vi "StoreArrays_V2.vi"(9 "Numeric":dbl, 10 "Value":u32[](array[numeric]), 11 "Value 2":i32[](array[numeric])) -> (3 "Cluster":cluster{"Value 2":i32[], "Value":u32[]})   [LabVIEW 2020]
uses:
  <vilib>/Utility/NIReport.llb/Report Type.ctl
  <vilib>/addons/_office/excel.llb/Excel Easy Table (str).vi
  <vilib>/Utility/NIReport.llb/NI_report.lvclass
  <vilib>/Utility/NIReport.llb/NI_ReportGenerationCore.lvlib
  <vilib>/Utility/NIReport.llb/Excel/NI_Excel.lvclass
  <vilib>/addons/_office/NI_ReportGenerationToolkit.lvlib
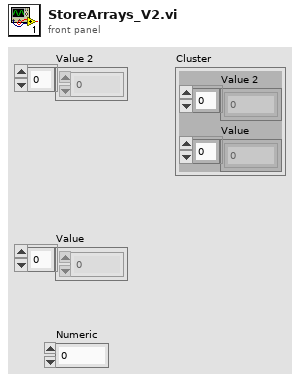
[diagram p1: front panel]
types:
  T1 = enum16{"open", "replace", "create", "open or create", "replace or create", "replace or create with confirmation"}
  T2 = typedef "NI_ReportGenerationCore.lvlib/Report Type.ctl" = enum16{"HTML", "Word", "Excel"}
  T3 = typedef "NI_Matrix.lvlib/RealMatrix.ctl" = dbl[][]
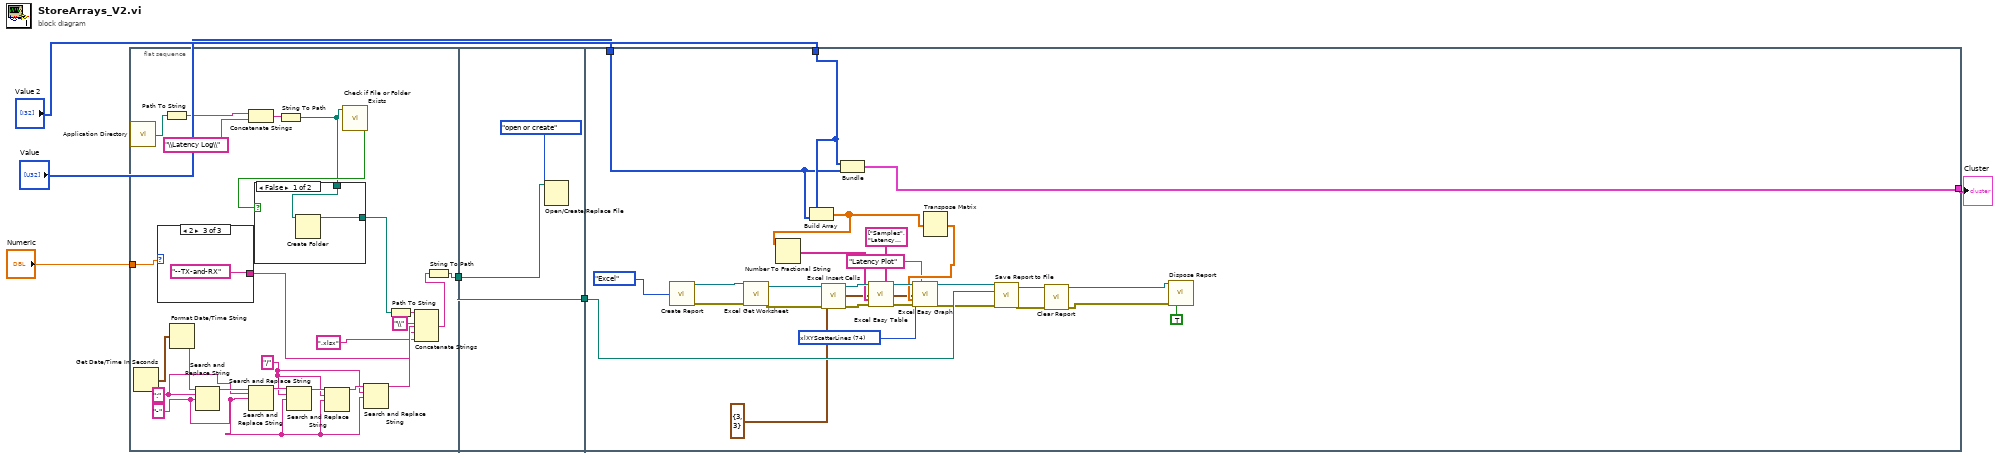
[diagram p0: block diagram]
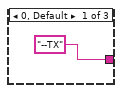
[diagram p2: hidden frame]
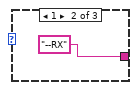
[diagram p3: hidden frame]
diagram:
  n1 = flat-sequence {
    tunnel: [w28] -> w6
    tunnel: "Numeric" -> [w8]
    tunnel: [w37] -> w5
    tunnel: w6 -> [w37]
    tunnel: w5 -> [w61]
    tunnel: "Value 2" -> [w55]
    tunnel: "Value" -> [w54]
    tunnel: [w56] -> w1
    frame #0 {
      w12 = "/" ("search string")
      w11 = "-" ("replace string (\"\")")
      w10 = ":" ("search string")
      n2 = call <vilib>:"Application Directory.vi"() -> ("Application Directory"=w25:path)
      n3 = Get Date/Time In Seconds() -> (seconds since 1Jan1904=w29:timestamp)
      n4 = case shown="2" w8 {
        tunnel: ["--TX" "--RX" "--TX-and-RX"] -> w7
        frame 0, Default {
        }
        frame 1 {
        }
        frame 2 {
        }
      }
      n5 = Path To String(path=w25) -> (string=w26:string)
      n6 = Format Date/Time String(seconds (now)=w29) -> (date/time string=w30:string)  [unwired: 2 in]
      n7 = Search and Replace String(input string=w30, search string=w10, replace string=w11) -> (result string=w17:string)  [unwired: 5 in, 3 out]
      n8 = Concatenate Strings(w26, "\\Latency Log\\" ("string")) -> (w23:string)
      n9 = Search and Replace String(input string=w17, search string=w10, replace string=w11) -> (result string=w16:string)  [unwired: 5 in, 3 out]
      n10 = String To Path(string=w23) -> (path=w19:path)
      n11 = Search and Replace String(input string=w16, search string=w12, replace string=w11) -> (result string=w15:string)  [unwired: 5 in, 3 out]
      n12 = Search and Replace String(input string=w15, search string=w12, replace string=w11) -> (result string=w14:string)  [unwired: 5 in, 3 out]
      n13 = call <vilib>:"Check if File or Folder Exists.vi"("path"=w19) -> ("file or folder exists?"=w22:bool)  [unwired: 8 in, 2 out]
      n14 = case shown="False" w22 {
        tunnel: [w35 w36] -> w20
        tunnel: w19 -> [w34 w36]
        frame False {
          n15 = Create Folder(path (use dialog)=w34) -> (created path=w35:path)  [unwired: 2 in, 2 out]
        }
        frame True {
        }
      }
      n16 = Search and Replace String(input string=w14, search string=w12, replace string=w11) -> (result string=w13:string)  [unwired: 5 in, 3 out]
      n17 = Path To String(path=w20) -> (string=w21:string)
      n18 = Concatenate Strings(w21, "\\" ("string"), w13, w7, ".xlsx" ("string")) -> (w27:string)
      n19 = String To Path(string=w27) -> (path=w28:path)
    }
    frame #1 {
      n20 = Open/Create/Replace File(file path (use dialog)=w37, operation (0:open)=T1."open or create") -> ()  [unwired: 4 in, 3 out]
    }
    frame #2 {
      w41 = 74 items=["xlColumnClustered"=51, "xlColumnStacked"=52, "xlColumnStacked100"=53, "xl3DColumnClustered"=54, "xl3DColumnStacked"=55, "xl3DColumnStacked100"=56, "xlBarClustered"=57, "xlBarStacked"=58, "xlBarStacked100"=59, "xl3DBarClustered"=60, "xl3DBarStacked"=61, "xl3DBarStacked100"=62, "xlLineStacked"=63, "xlLineStacked100"=64, "xlLineMarkers"=65, "xlLineMarkersStacked"=66, "xlLineMarkersStacked100"=67, "xlPieOfPie"=68, "xlPieExploded"=69, "xl3DPieExploded"=70, "xlBarOfPie"=71, "xlXYScatterSmooth"=72, "xlXYScatterSmoothNoMarkers"=73, "xlXYScatterLines"=74, "xlXYScatterLinesNoMarkers"=75, "xlAreaStacked"=76, "xlAreaStacked100"=77, "xl3DAreaStacked"=78, "xl3DAreaStacked100"=79, "xlDoughnutExploded"=80, "xlRadarMarkers"=81, "xlRadarFilled"=82, "xlSurface"=83, "xlSurfaceWireframe"=84, "xlSurfaceTopView"=85, "xlSurfaceTopViewWireframe"=86, "xlBubble"=15, "xlBubble3DEffect"=87, "xlStockHLC"=88, "xlStockOHLC"=89, "xlStockVHLC"=90, "xlStockVOHLC"=91, "xlCylinderColClustered"=92, "xlCylinderColStacked"=93, "xlCylinderColStacked100"=94, "xlCylinderBarClustered"=95, "xlCylinderBarStacked"=96, "xlCylinderBarStacked100"=97, "xlCylinderCol"=98, "xlConeColClustered"=99, "xlConeColStacked"=100, "xlConeColStacked100"=101, "xlConeBarClustered"=102, "xlConeBarStacked"=103, "xlConeBarStacked100"=104, "xlConeCol"=105, "xlPyramidColClustered"=106, "xlPyramidColStacked"=107, "xlPyramidColStacked100"=108, "xlPyramidBarClustered"=109, "xlPyramidBarStacked"=110, "xlPyramidBarStacked100"=111, "xlPyramidCol"=112, "xl3DColumn"=-4100, "xlLine"=4, "xl3DLine"=-4101, "xl3DPie"=-4102, "xlPie"=5, "xlXYScatter"=-4169, "xl3DArea"=-4098, "xlArea"=1, "xlDoughnut"=-4120, "xlRadar"=-4151] ("graph type (col clustered)")
      n21 = call <vilib>:"Create Report.vi"("report type"=Report_Type."Excel") -> ("report out"=w64:refnum<class "NI_report.lvclass">, "error out"=w63:errorcluster)  [unwired: 13 in]
      n22 = call <vilib>:"Excel Get Worksheet.vi"("report in"=w64, "error in (no error)"=w63) -> ("report out"=w49:refnum<class "NI_report.lvclass">, "error out"=w48:errorcluster)  [unwired: 12 in]
      n23 = Build Array(w55, w54) -> (w43:T3)
      n24 = Number To Fractional String(number=w43) -> (F-format string=w50:string[][])  [unwired: 3 in]
      n25 = call <vilib>:"Excel Insert Cells.vi"("report in"=w49, "error in (no error)"=w48) -> ("report out"=w53:refnum<class "NI_report.lvclass">, "error out"=w52:errorcluster)  [unwired: 12 in]
      n26 = Bundle("Value 2"=w55, "Value"=w54) -> (w56:cluster{"Value 2":i32[], "Value":u32[]})  [unwired: 1 in]
      n27 = call-poly <vilib>:"Excel Easy Table.vi"("report in"=w53, "text data"=w50, "error in (no error)"=w52, "column headers"=string[] ["Samples", "Latency (ms)"]) -> ("report out"=w47:refnum<class "NI_report.lvclass">, "error out"=w46:errorcluster)  [unwired: 7 in, 3 out]
      n28 = Transpose Matrix(1:w43) -> (0:w42:T3)
      n29 = call <vilib>:"Excel Easy Graph.vi"("report in"=w47, "graph title (\"\")"="Latency Plot" ("graph title (\"\")"), "graph type (col clustered)"=w41, "start (0, 0)"=cluster{"row":i32, "column":i32} {"row"=3, "column"=3}, "data"=w42, "error in (no error)"=w46) -> ("report out"=w45:refnum<class "NI_report.lvclass">, "error out"=w44:errorcluster)  [unwired: 8 in]
      n30 = call-dynamic "Save Report to File.vi"("report in"=w45, "report file path"=w61, "error in (no error)"=w44) -> ("report out"=w60:refnum<class "NI_report.lvclass">, "error out"=w59:errorcluster)  [unwired: 11 in]
      n31 = call-dynamic "Clear Report.vi"("report in"=w60, "error in (no error)"=w59) -> ("report out"=w58:refnum<class "NI_report.lvclass">, "error out"=w57:errorcluster)  [unwired: 12 in]
      n32 = call-dynamic "Dispose Report.vi"("report in"=w58, "error in (no error)"=w57, "close report? (T)"=TRUE) -> ()  [unwired: 12 in, 1 out]
    }
  }
  "Cluster" <- w1
